vi "Extract Peak-Peak Voltage.vi"(0 "Input Waveform":T1, 1 "Frequency (Hz)":dbl, 2 "Search %":dbl, 5 "Output Waveform":T1, 9 "Actual Sample Rate":dbl, 11 "error in (no error)":errorcluster) -> (4 "Detected Output Voltage":dbl, 6 "Detected Input Voltage":dbl, 15 "error out":errorcluster)   [LabVIEW 2020, in "LDO PSRR.lvlib"]
uses:
  LDO PSRR.lvlib
  <vilib>/measure/matone.llb/Extract Single Tone Information 1 Chan.vi
  <vilib>/measure/NI_MAPro.lvlib
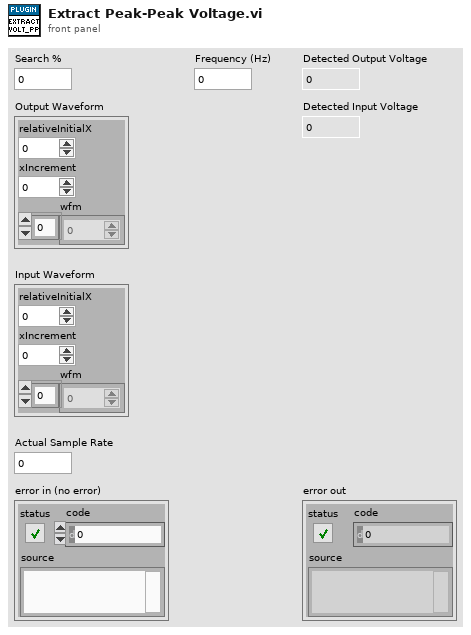
[diagram p1: front panel]
types:
  T1 = cluster{"relativeInitialX":dbl, "xIncrement":dbl, "wfm":dbl[]}
  T2 = cluster{"approx freq. (optional)":dbl, "search (+/- % of Fsampl.)":dbl}
  T3 = enum32{"none", "input signal", "detected signal", "residual signal"}
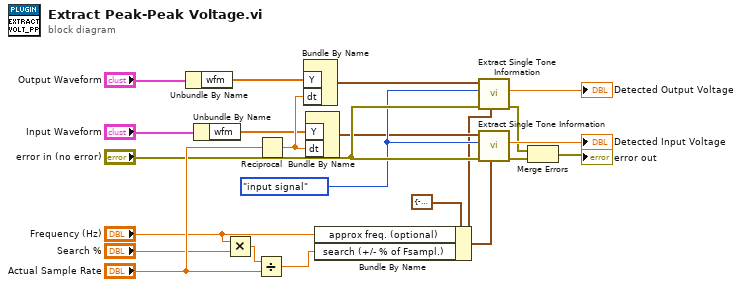
[diagram p0: block diagram]
diagram:
  w14 = T3."input signal" ("export mode")
  n1 = Unbundle By Name("Output Waveform") -> ("wfm"=w9:dbl[])
  n2 = Unbundle By Name("Input Waveform") -> ("wfm"=w8:dbl[])
  n3 = Multiply(x="Frequency (Hz)", y="Search %") -> (x*y=w3:dbl)
  n4 = Divide(x=w3, y="Actual Sample Rate") -> (x/y=w2:dbl)
  n5 = Reciprocal(x="Actual Sample Rate") -> (1/x=w12:dbl)
  n6 = Bundle By Name("Y"=w9, "dt"=w12) -> (w1:waveform(dbl))  [unwired: 1 in]
  n7 = Bundle By Name("Y"=w8, "dt"=w12) -> (w11:waveform(dbl))  [unwired: 1 in]
  n8 = Bundle By Name(cluster=T2 {"approx freq. (optional)"=-1.0, "search (+/- % of Fsampl.)"=5.0} ("Set Frequency(Hz)"), "approx freq. (optional)"="Frequency (Hz)", "search (+/- % of Fsampl.)"=w2) -> (w10:T2)
  n9 = call-poly <vilib>:"Extract Single Tone Information.vi"("advanced search"=w10, "error in (no error)"="error in (no error)", "export mode"=w14, "time signal in"=w1) -> ("error out"=w6:errorcluster, "detected amplitude"=→"Detected Output Voltage":dbl)  [unwired: 2 in, 4 out]
  n10 = call-poly <vilib>:"Extract Single Tone Information.vi"("advanced search"=w10, "error in (no error)"="error in (no error)", "export mode"=w14, "time signal in"=w11) -> ("error out"=w7:errorcluster, "detected amplitude"=→"Detected Input Voltage":dbl)  [unwired: 2 in, 4 out]
  n11 = Merge Errors(w6, w7) -> (→"error out":errorcluster)
